vi "Get List Variable.vi"(8 "error in (no error)":errorcluster, 11 "VI in":refnum<vi>) -> (3 "Array":string[][](array[string]))   [LabVIEW 2019]
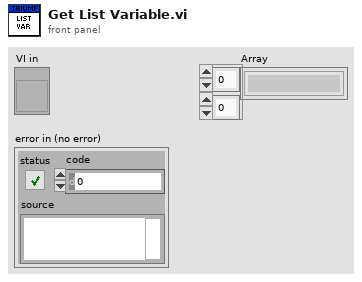
[diagram p1: front panel]
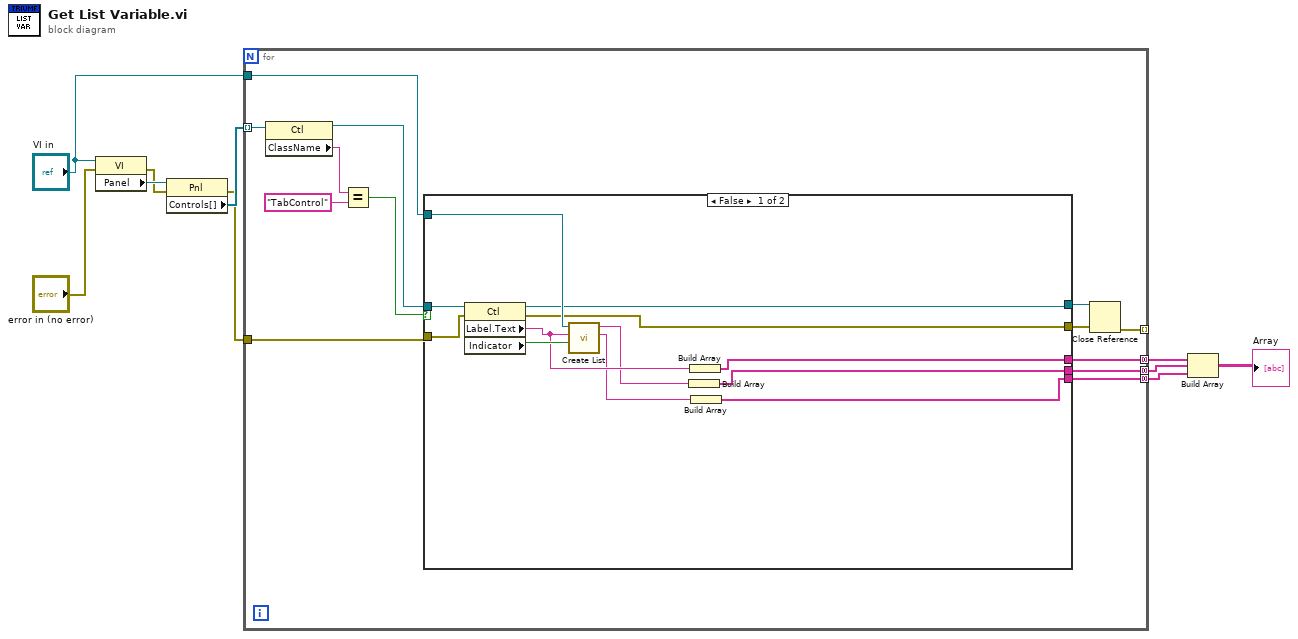
[diagram p0: block diagram]
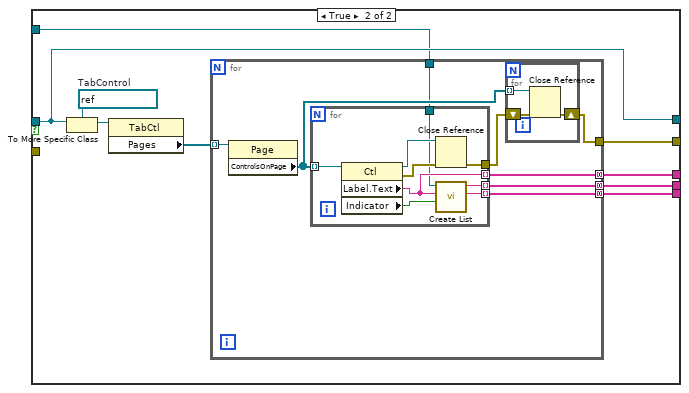
[diagram p2: hidden frame]
diagram:
  n1 = property class="VI"(reference="VI in", error in="error in (no error)") -> (error out=w6:errorcluster, "Panel"=w7:refnum<vi>)  [unwired: 1 out]
  n2 = property class="Pnl"(reference=w7, error in=w6) -> (error out=w5:errorcluster, "Controls[]"=w8:refnum<vi>[])  [unwired: 1 out]
  n3 = for {
    tunnel: w8 -> [w23] mode=indexing
    tunnel: "VI in" -> [w16]
    tunnel: [w17] -> _ mode=indexing
    tunnel: w5 -> [w15]
    tunnel: [w14] -> w4 mode=concatenating
    tunnel: [w13] -> w3 mode=concatenating
    tunnel: [w12] -> w2 mode=concatenating
    n4 = property class="Ctl"(reference=w23) -> (reference out=w21:refnum<vi>, "ClassName"=w11:string)  [unwired: 1 in, 1 out]
    n5 = Equal?(x=w11, y="TabControl") -> (x = y?=w20:bool)
    n6 = case shown="False" w20 {
      tunnel: w21 -> [w35 w40]
      tunnel: [w30 w41] -> w19
      tunnel: [w31 w40] -> w18
      tunnel: w16 -> [w32 w39]
      tunnel: w15 -> [w34 _]
      tunnel: [w26 w38] -> w14
      tunnel: [w25 w37] -> w13
      tunnel: [w24 w36] -> w12
      frame False {
        n7 = property class="Ctl"(reference=w35, error in=w34) -> (reference out=w31:refnum<vi>, error out=w30:errorcluster, "Label.Text"=w29:string, "Indicator"=w33:bool)
        n8 = call "Create List.vi"("Indicator"=w33, "Label.Text"=w29, "VI in"=w32) -> ("format string"=w27:string, "String"=w28:string)  [unwired: 7 in]
        n9 = Build Array(w28) -> (w25:string[])
        n10 = Build Array(w29) -> (w26:string[])
        n11 = Build Array(w27) -> (w24:string[])
      }
      frame True {
        w43 = refnum<vi> refnum  # TabControl
        n12 = To More Specific Class(target class=w43, reference=w40) -> (specific class reference=w44:refnum<vi>)  [unwired: 1 in, 1 out]
        n13 = property class="TabCtl"(reference=w44) -> ("Pages"=w42:refnum<vi>[])  [unwired: 1 in, 2 out]
        n14 = for {
          tunnel: w42 -> [w52] mode=indexing
          tunnel: [w49] -> w41
          tunnel: w39 -> [w48]
          tunnel: [w47] -> w38 mode=concatenating
          tunnel: [w46] -> w37 mode=concatenating
          tunnel: [w45] -> w36 mode=concatenating
          n15 = property class="Page"(reference=w52) -> ("ControlsOnPage"=w51:refnum<vi>[])  [unwired: 1 in, 2 out]
          n16 = for {
            tunnel: w51 -> [w64] mode=indexing
            tunnel: [w62] -> w45 mode=indexing
            tunnel: [w61] -> w46 mode=indexing
            tunnel: [w60] -> w47 mode=indexing
            tunnel: [w57] -> w50
            tunnel: w48 -> [w56]
            n17 = property class="Ctl"(reference=w64) -> (reference out=w58:refnum<vi>, error out=w59:errorcluster, "Label.Text"=w60:string, "Indicator"=w63:bool)  [unwired: 1 in]
            n18 = Close Reference(reference=w58, error in (no error)=w59) -> (error out=w57:errorcluster)
            n19 = call "Create List.vi"("Indicator"=w63, "Label.Text"=w60, "VI in"=w56) -> ("format string"=w62:string, "String"=w61:string)  [unwired: 7 in]
          }
          n20 = for {
            tunnel: w51 -> [w55] mode=indexing
            shift-right: [w54] -> w49
            shift-left: w50 -> [w53]
            n21 = Close Reference(reference=w55, error in (no error)=w53) -> (error out=w54:errorcluster)
          }
        }
      }
    }
    n22 = Close Reference(reference=w18, error in (no error)=w19) -> (error out=w17:errorcluster)
  }
  n23 = Build Array(w4, w3, w2) -> (→"Array":string[][])
